vi "环境参数数据插入.vi"(0 "data":T1, 3 "错误输入（无错误）":errorcluster, 4 "数据库类型":T2) -> (10 "错误输出":errorcluster)   [LabVIEW 2016]
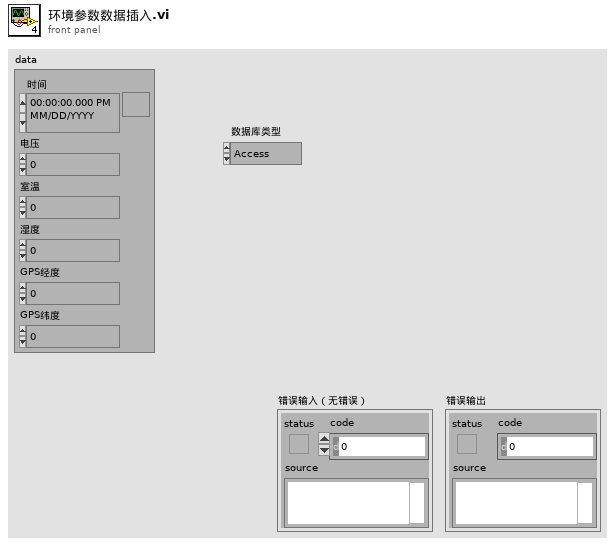
[diagram p1: front panel]
types:
  T1 = cluster{"时间":timestamp, "电压":dbl, "室温":dbl, "湿度":dbl, "GPS经度":dbl, "GPS纬度":dbl}
  T2 = typedef "数据库类型.ctl" = enum16{"Access", "SQLite"}
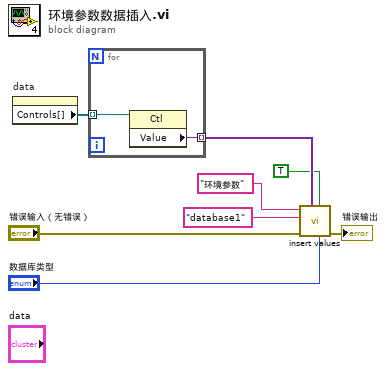
[diagram p0: block diagram]
diagram:
  n1 = property on="data" class="Clust (严格)"() -> ("Controls[]"=w2:refnum<vi>[])  [unwired: 2 in, 2 out]
  n2 = for {
    tunnel: w2 -> [w10] mode=indexing
    tunnel: [w9] -> w8 mode=indexing
    n3 = property class="Ctl"(reference=w10) -> ("Value"=w9:variant)  [unwired: 1 in, 2 out]
  }
  n4 = call "insert values.vi"("数据库类型"="数据库类型", "是否创建唯一键"=TRUE, "data"=w8, "错误输入（无错误）"="错误输入（无错误）", "database"="database1", "Tabe Name"="环境参数" ("table")) -> ("错误输出"=→"错误输出":errorcluster)  [unwired: 5 in]
